vi "Add Digital Output Channels.vi"(8 "error in (no error)":errorcluster, 9 "DIO Port Settings":T1[](array[typedef]), 11 "DAQ Ref":refnum<k24>) -> (0 "error out":errorcluster, 3 "DAQ Ref":refnum<k24>)   [LabVIEW 2019, in "Simple SysDef API.lvlib"]
uses:
  <userlib>/SimpleSysDef/Simple SysDef API.lvlib
  NationalInstruments.VeriStand.SystemDefinitionAPI
  <userlib>/SimpleSysDef/_SubVIs/Add DAQ Hardware_Digital Port Settings.ctl
  <userlib>/SimpleSysDef/_SubVIs/Add DAQ Hardware_Digital Settings.ctl
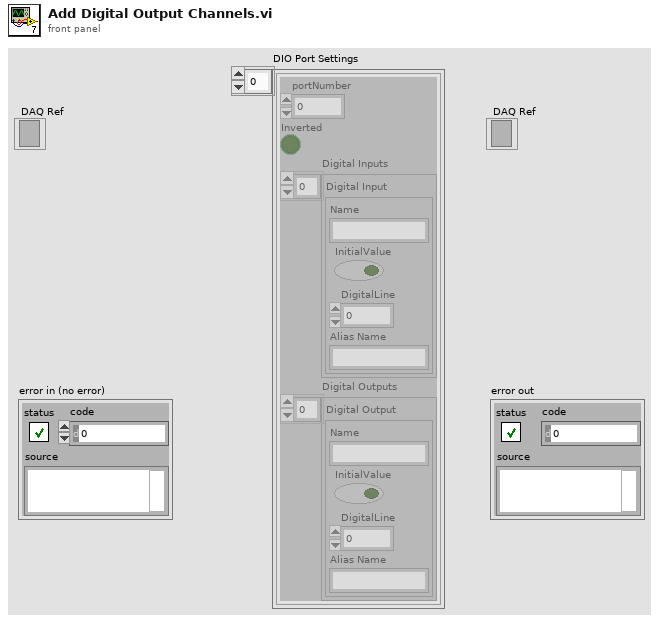
[diagram p1: front panel]
types:
  T1 = typedef "Simple SysDef API.lvlib/Add DAQ Hardware_Digital Port Settings.ctl" = cluster{"portNumber":u32, "Inverted":bool, "Digital Inputs":T2[], "Digital Outputs":T2[]}
  T2 = typedef "Simple SysDef API.lvlib/Add DAQ Hardware_Digital Settings.ctl" = cluster{"Name":string, "InitialValue":bool, "DigitalLine":u32, "Alias Name":string}
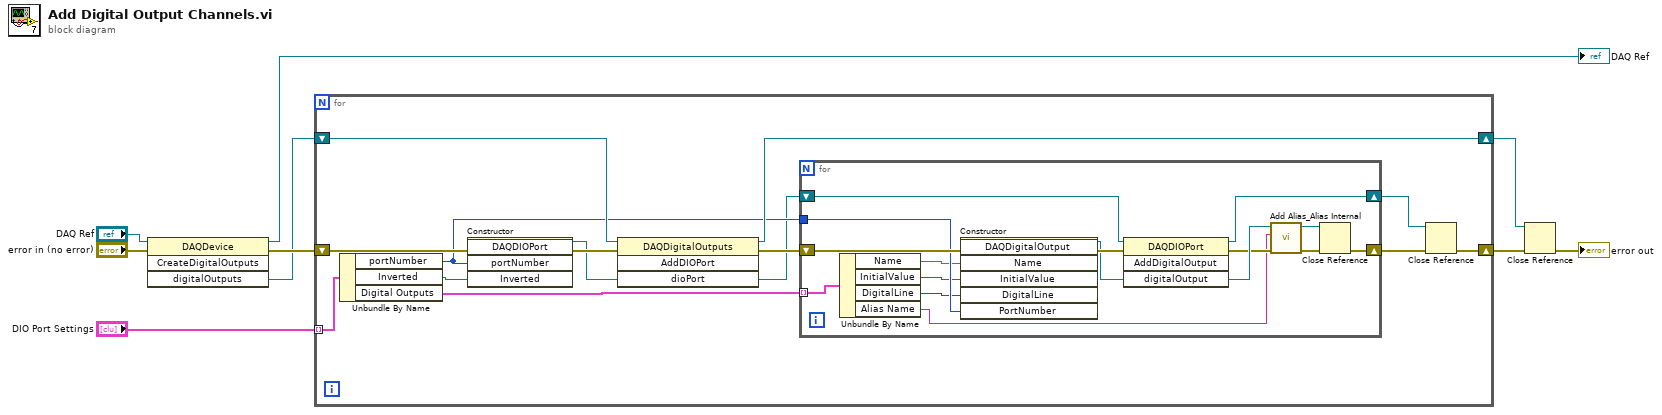
[diagram p0: block diagram]
diagram:
  n1 = invoke class="DAQDevice" method="CreateDigitalOutputs"(reference="DAQ Ref", error in="error in (no error)") -> (reference out=→"DAQ Ref":refnum<k24>, error out=w4:errorcluster, "digitalOutputs"=w1:refnum<k24>)  [unwired: 2 in, 1 out]
  n2 = for {
    shift-right: [w20] -> w6
    shift-left: w4 -> [w21]
    shift-right: [w19] -> w7
    shift-left: w1 -> [w22]
    tunnel: "DIO Port Settings" -> [w16] mode=indexing
    n3 = Unbundle By Name(w16) -> ("portNumber"=w17:u32, "Inverted"=w18:bool, "Digital Outputs"=w15:T2[])
    n4 = constructor class="DAQDIOPort"(error in=w21, "portNumber"=w17, "Inverted"=w18) -> (reference out=w10:refnum<k24>, error out=w11:errorcluster)  [unwired: 2 in, 3 out]
    n5 = invoke class="DAQDigitalOutputs" method="AddDIOPort"(reference=w22, error in=w11, "dioPort"=w10) -> (reference out=w19:refnum<k24>, error out=w12:errorcluster)  [unwired: 1 in, 2 out]
    n6 = for {
      shift-right: [w33] -> w13
      shift-left: w12 -> [w35]
      shift-right: [w36] -> w14
      shift-left: w10 -> [w37]
      tunnel: w17 -> [w32]
      tunnel: w15 -> [w31] mode=indexing
      n7 = Unbundle By Name(w31) -> ("Name"=w28:string, "InitialValue"=w29:bool, "DigitalLine"=w30:u32, "Alias Name"=w23:string)
      n8 = constructor class="DAQDigitalOutput"(error in=w35, "Name"=w28, "InitialValue"=w29, "DigitalLine"=w30, "PortNumber"=w32) -> (reference out=w27:refnum<k24>, error out=w34:errorcluster)  [unwired: 2 in, 5 out]
      n9 = invoke class="DAQDIOPort" method="AddDigitalOutput"(reference=w37, error in=w34, "digitalOutput"=w27) -> (reference out=w36:refnum<k24>, error out=w25:errorcluster)  [unwired: 1 in, 2 out]
      n10 = call <userlib>:"Add Alias_Alias Internal.vi"("error in (no error)"=w25, "Name"=w23, "Base Node"=w27) -> ("error out"=w24:errorcluster, "Base Node out"=w26:refnum<k24>)  [unwired: 7 in]
      n11 = Close Reference(reference=w26, error in (no error)=w24) -> (error out=w33:errorcluster)
    }
    n12 = Close Reference(reference=w14, error in (no error)=w13) -> (error out=w20:errorcluster)
  }
  n13 = Close Reference(reference=w7, error in (no error)=w6) -> (error out=→"error out":errorcluster)
